vi "stackDump.vi"(8 "error in (no error)":errorcluster, 11 "lua_state_p":u64) -> (0 "error out":errorcluster, 2 "stack":string[](array[string]), 3 "lua_state_p out":u64)   [LabVIEW 2020, in "lua.dll.lvlib"]
uses:
  lua.dll.lvlib
  lua_types.ctl
  lua_typename.vi
  lua_tolstring.vi
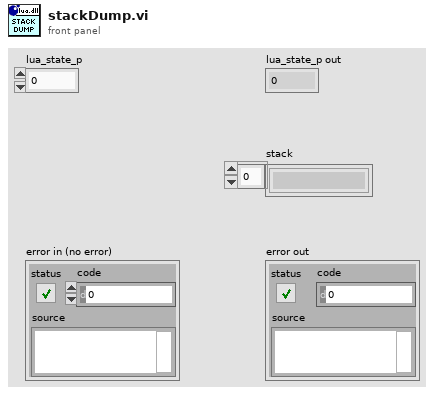
[diagram p1: front panel]
types:
  T1 = typedef "lua.dll.lvlib/lua_types.ctl" = i32
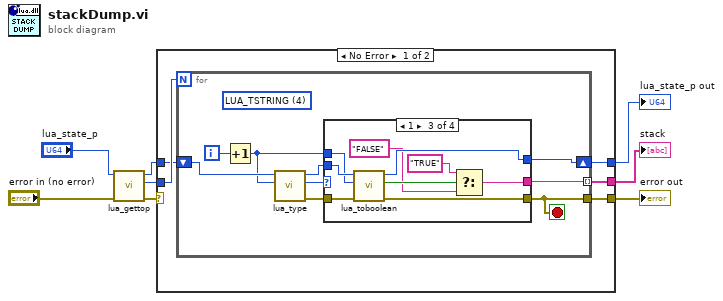
[diagram p0: block diagram]
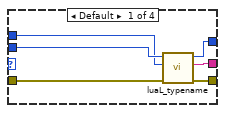
[diagram p2: hidden frame]
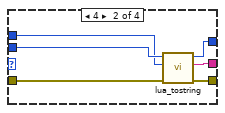
[diagram p3: hidden frame]
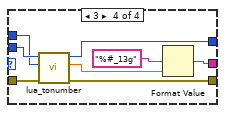
[diagram p4: hidden frame]
diagram:
  n1 = call "lua_gettop.vi"("error in (no error)"="error in (no error)", "lua_state_p"="lua_state_p") -> ("error out"=w4:errorcluster, "index"=w6:i32, "lua_state_p out"=w5:u64)  [unwired: 7 in]
  n2 = case shown="No Error" w4 {
    selector: w4 -> [_ w53]
    tunnel: w6 -> [w13 _]
    tunnel: w5 -> [w12 w52]
    tunnel: [w10 w53] -> w3
    tunnel: [w11 w52] -> w2
    tunnel: [w9 _] -> w1
    frame No Error {
      n3 = for {
        N: w13 -> [_]
        shift-right: [w17] -> w11
        shift-left: w12 -> [w21]
        tunnel: [w15] -> w10
        tunnel: [w19] -> w9 mode=indexing
        i -> [w22]
        stop <- w15 stop-if-true
        (unwired) T1 4 items=["LUA_TNONE"=-1, "LUA_TNIL"=0, "LUA_TBOOLEAN"=1, "LUA_TLIGHTUSERDATA"=2, "LUA_TNUMBER"=3, "LUA_TSTRING"=4, "LUA_TTABLE"=5, "LUA_TFUNCTION"=6, "LUA_TUSERDATA"=7, "LUA_TTHREAD"=8, "LUA_NUMTYPES"=9] ("lua type")
        n4 = Increment(x=w22) -> (x+1=w14:i32)
        n5 = call "lua_type.vi"("index"=w14, "lua_state_p"=w21) -> ("error out"=w16:errorcluster, "lua type"=w20:T1, "lua_state_p out"=w18:u64)  [unwired: 7 in]
        n6 = case shown="1" w20 {
          tunnel: [w25 w29 w35 w45] -> w19
          tunnel: w18 -> [w28 w34 w43 w51]
          tunnel: [w27 w33 w42 w50] -> w17
          tunnel: w16 -> [w23 w32 w41 w49]
          tunnel: [w26 w31 w40 w48] -> w15
          tunnel: w14 -> [w24 w30 w39 w47]
          frame Default {
            n7 = call "luaL_typename.vi"("error in (no error)"=w23, "index"=w24, "lua_state_p"=w28) -> ("error out"=w26:errorcluster, "string"=w25:string, "lua_state_p out"=w27:u64)  [unwired: 6 in]
          }
          frame 4 {
            n8 = call "lua_tostring.vi"("error in (no error)"=w32, "index"=w30, "lua_state_p"=w34) -> ("error out"=w31:errorcluster, "string"=w29:string, "lua_state_p out"=w33:u64)  [unwired: 6 in]
          }
          frame 1 {
            n9 = call "lua_toboolean.vi"("error in (no error)"=w41, "index"=w39, "lua_state_p"=w43) -> ("error out"=w40:errorcluster, "boolean"=w38:bool, "lua_state_p out"=w42:u64)  [unwired: 6 in]
            n10 = Select(t="TRUE", s=w38, f="FALSE") -> (s? t:f=w35:string)
          }
          frame 3 {
            n11 = call "lua_tonumber.vi"("error in (no error)"=w49, "index"=w47, "lua_state_p"=w51) -> ("error out"=w48:errorcluster, "number"=w44:dbl, "lua_state_p out"=w50:u64)  [unwired: 5 in, 1 out]
            n12 = Format Value(format string="%#_13g", value (0)=w44) -> (output string=w45:string)  [unwired: 1 in]
          }
        }
      }
    }
    frame Error {
    }
  }
  "error out" <- w3
  "lua_state_p out" <- w2
  "stack" <- w1
